vi "Append First Packet 26_01_18.vi"(4 "Movement Correction":bool, 6 "Repeat Scan":i32, 7 "MAC Address":string, 8 "Ny":i32, 9 "Nx":i32, 10 "Packets":string[](array[string]), 11 "AOL_Globals":T1={"Imaging Protocol"=enum."AOL Z-Stack", "Number of POI"=0, "Number of Miniscans"=0, "Number of Trials"=0, "Number of Cycles "=0, "# Averaged Frames"=0, "Laser power (%)"=0, "Pockels (V)"=0.0, "Acquisition Length (sec)"=0.0, "Fill time (us)"=0.0, "POI Dwell time (us)"=0.0, "Miniscan Dwell time per pixel (us)"=0.0, "PMT 1"=0.0, "PMT 2"=0.0, "Back Apperture (mA)"=0.0, "Frame Size"=0, "Center Frequency"=0.0, "Field of View (norm)"=0.0, "DwellTime (us)"=0.0, "Wavelength (nm)"=0.0, "Zoom"=0.0, "AOL Z"=0.0, "AOL Mode"=enum."Raster", "GridXY"=0.0, "GridZ"=0.0, "TriggerPeriod (sec)"=0.0, "Number of Pixels in Miniscan"=0, "Experiment folder path"=path "", "X centre"=0.0, "Y centre"=0.0, "Angle (degrees)"=0.0, "Plane Mode"=0, "Threshold"=[], "Regenerate Chirps"=FALSE, "Rectangle ROI length (pixels)"=0, "Rectangle ROI height (pixels)"=0, "AOD fill"=4900, "StartupDelay"=0, "Samples Wait after Trigger"=5080, "Slip Cycle"=600000, "Add Cycle"=TRUE, "Functional Mode"=enum."Point", "Z Start"=0.0, "Z Stop"=0.0, "# Planes"=0, "Total Pixels"=0, "Variable Miniscan Pixels"=[], "Use Variable Length"=FALSE, "Use Variable Resolution"=FALSE, "Laser power (%) at Z Start"=0, "Laser power (%) at Z Stop"=0, "Ref Z Step"=0, "Ref Dwell Time (us)"=0.0, "Field of View (um)"=175.0} {"Plane Mode" items=["XY Plane", "XZ Plane", "YZ Plane", "arbitraryplane"]; "Frame Size" items=["100X100"=100, "128X128"=128, "200X200"=200, "256X256"=256, "512X512"=512, "1024x1024"=1024, "2048x2048"=2048]; "Back Apperture (mA)" format="%#.6g"; "Pockels (V)" format="%#.6g"; "PMT 2" format="%#.6g"; "PMT 1" format="%#.6g"; "Angle (degrees)" format="%#.6g"; "POI Dwell time (us)" format="%#.6g"}) -> (0 "Repeat":i32, 2 "HexPackets":string[](array[string]), 3 "Total Packets":i32)   [LabVIEW 2020]
uses:
  Typedefs/Imaging Protocols enum.ctl
  Typedefs/Controls/AOL_Globals.ctl
  Typedefs/AOL modes.ctl
  Typedefs/Plane Mode.ctl
  Typedefs/Frame Size.ctl
  Typedefs/Functional Mode.ctl
panel:
  # "RE-ENTRANT"
  # "SUB-ROUTINE"
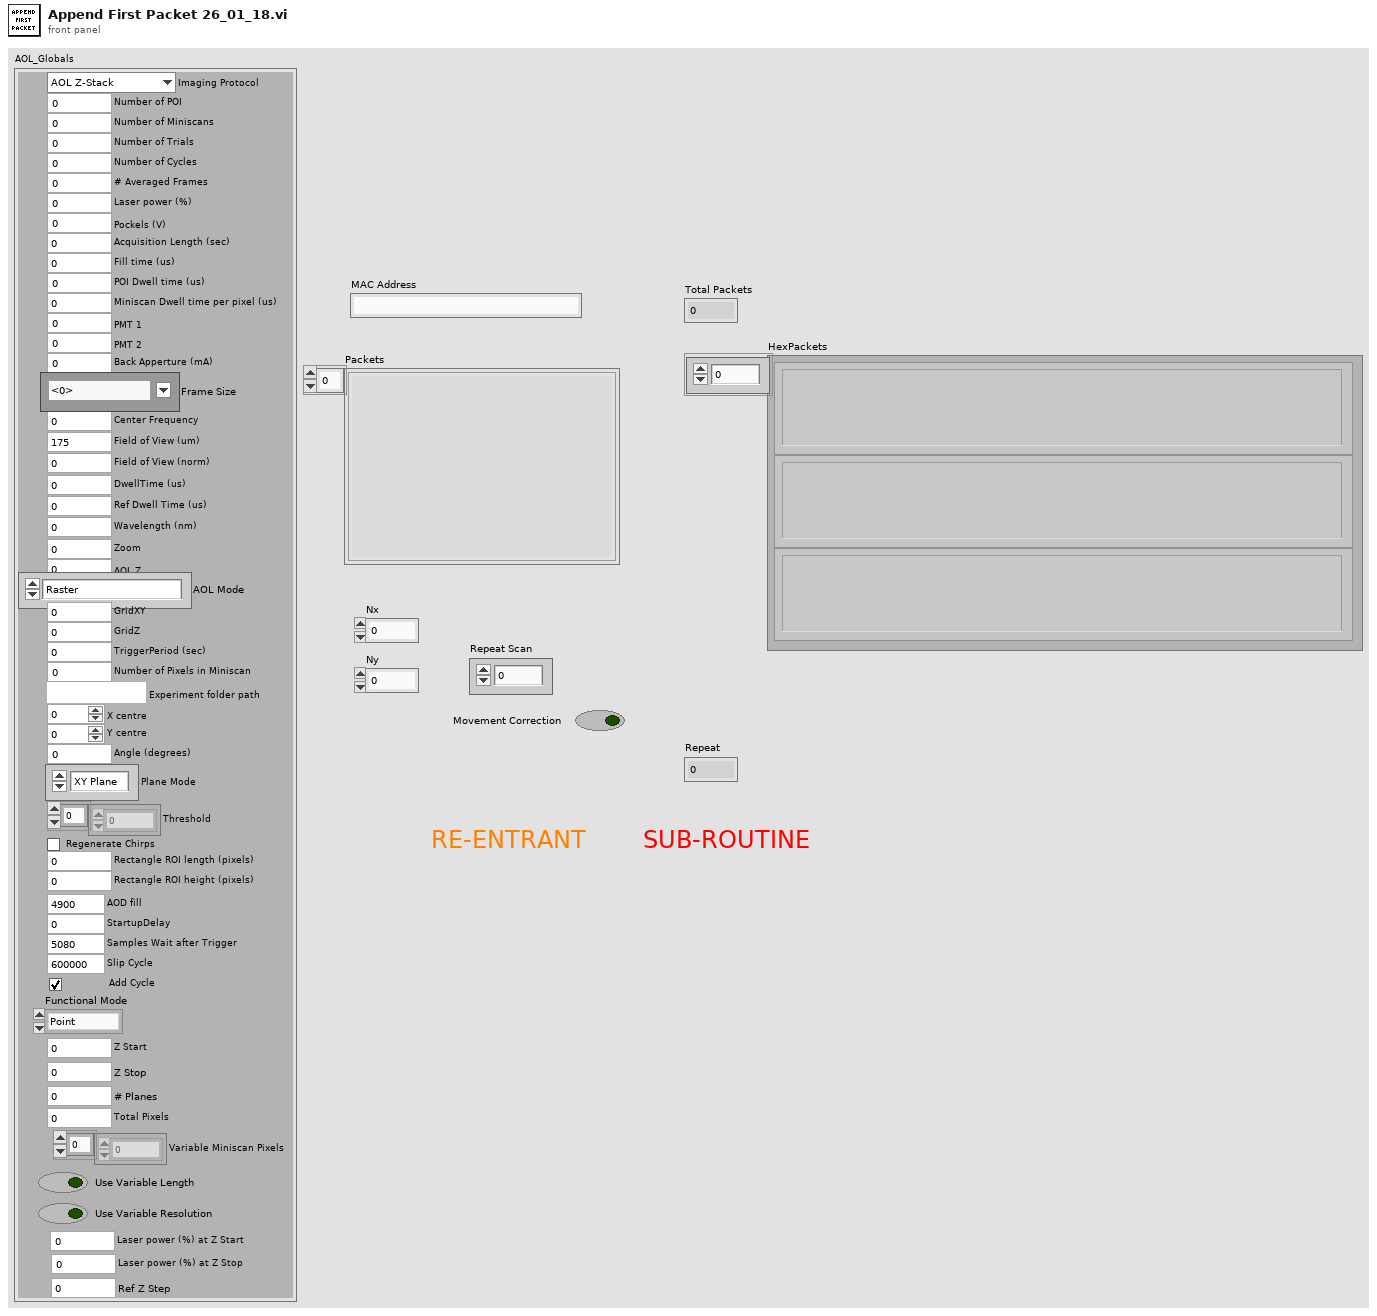
[diagram p1: front panel]
types:
  T1 = typedef "AOL_Globals.ctl" = cluster{"Imaging Protocol":T2, "Number of POI":u16, "Number of Miniscans":u16, "Number of Trials":u16, "Number of Cycles ":u64, "# Averaged Frames":u16, "Laser power (%)":u8, "Pockels (V)":dbl, "Acquisition Length (sec)":dbl, "Fill time (us)":dbl, "POI Dwell time (us)":dbl, "Miniscan Dwell time per pixel (us)":dbl, "PMT 1":dbl, "PMT 2":dbl, "Back Apperture (mA)":dbl, "Frame Size":T3, "Center Frequency":dbl, "Field of View (norm)":dbl, "DwellTime (us)":dbl, "Wavelength (nm)":dbl, "Zoom":dbl, "AOL Z":dbl, "AOL Mode":T4, "GridXY":dbl, "GridZ":dbl, "TriggerPeriod (sec)":dbl, "Number of Pixels in Miniscan":u16, "Experiment folder path":path, "X centre":dbl, "Y centre":dbl, "Angle (degrees)":dbl, "Plane Mode":T5, "Threshold":u16[], "Regenerate Chirps":bool, "Rectangle ROI length (pixels)":u16, "Rectangle ROI height (pixels)":u16, "AOD fill":u16, "StartupDelay":i32, "Samples Wait after Trigger":u16, "Slip Cycle":u32, "Add Cycle":bool, "Functional Mode":T6, "Z Start":dbl, "Z Stop":dbl, "# Planes":i32, "Total Pixels":i32, "Variable Miniscan Pixels":u16[], "Use Variable Length":bool, "Use Variable Resolution":bool, "Laser power (%) at Z Start":u8, "Laser power (%) at Z Stop":u8, "Ref Z Step":i8, "Ref Dwell Time (us)":dbl, "Field of View (um)":dbl}
  T2 = typedef "Imaging Protocols enum.ctl" = enum16{"AOL Z-Stack", "Motor Z Stack", "Functional Acquisition", "Single Plane Acquisition", "Volume Acquisition", "Live Imaging", "Live Plane Imaging", "Live Volume Imaging"}
  T3 = typedef "Frame Size.ctl" = u16
  T4 = typedef "AOL modes.ctl" = enum16{"Raster", "Structural", "Pointing", "Mini Scan", "Alignment"}
  T5 = typedef "Plane Mode.ctl" = u16
  T6 = typedef "Functional Mode.ctl" = enum16{"Point", "Line", "Patch", "Plane", "Volume"}
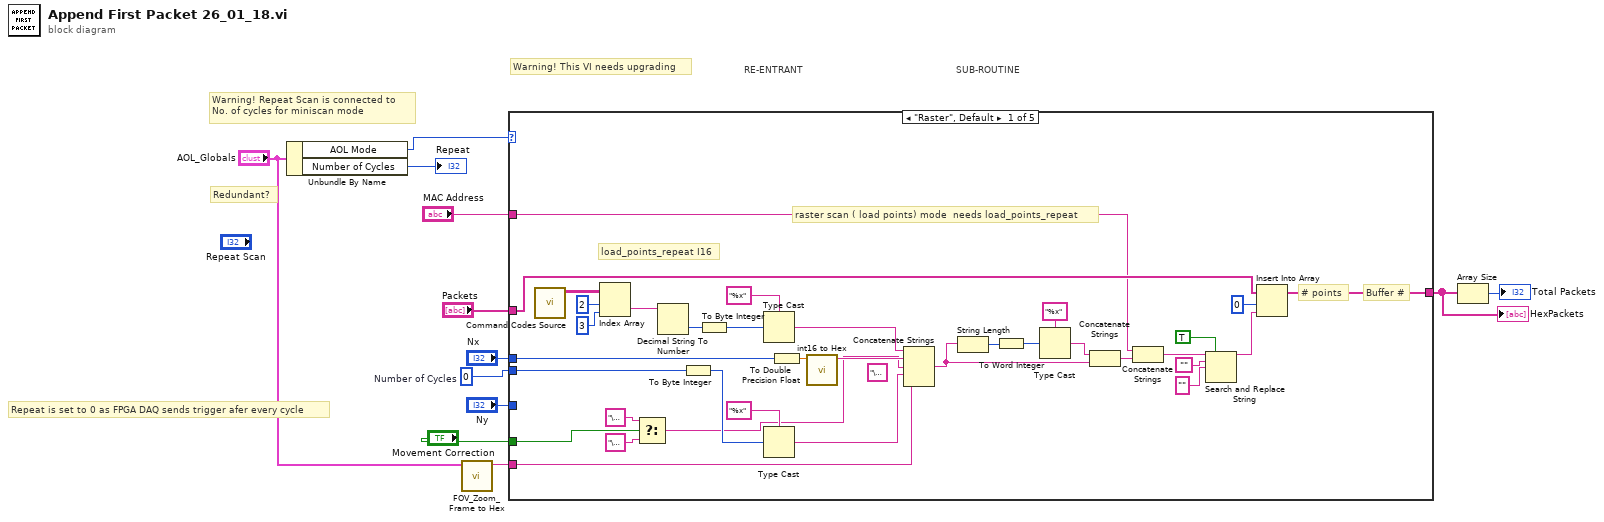
[diagram p0: block diagram]
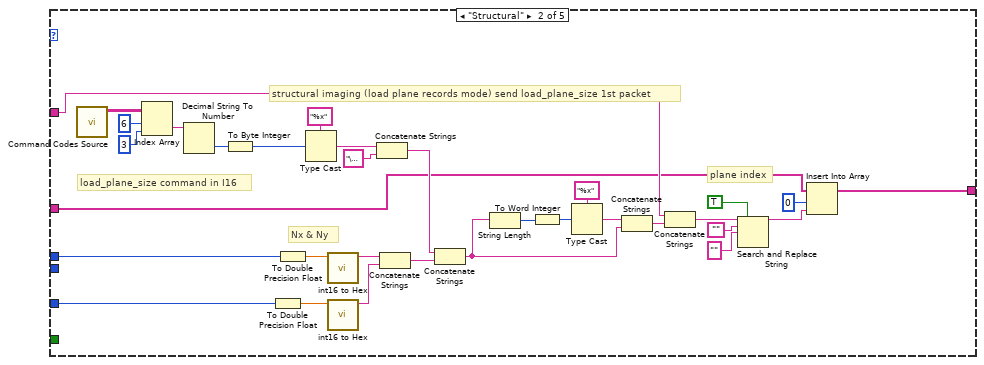
[diagram p2: hidden frame]
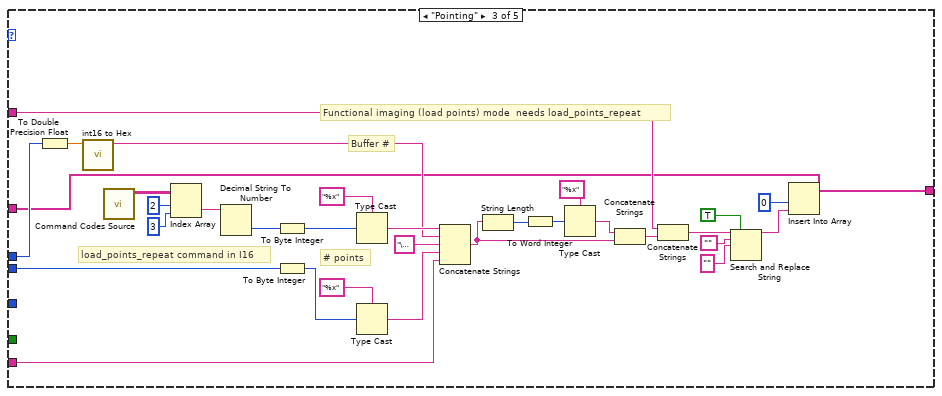
[diagram p3: hidden frame]
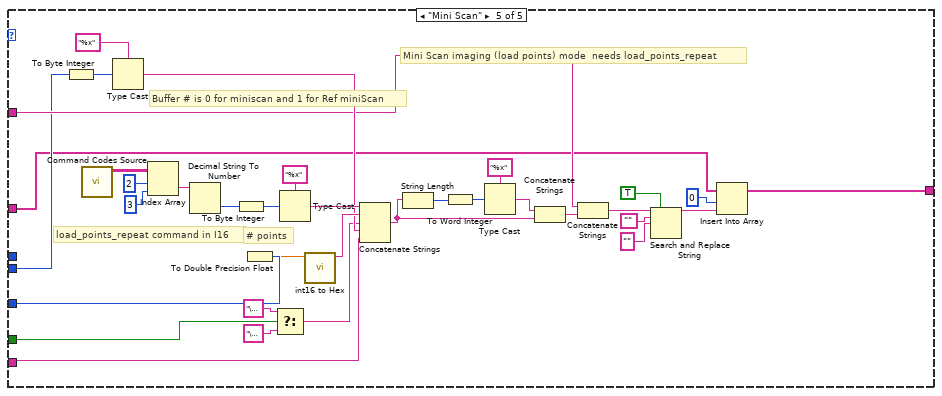
[diagram p5: hidden frame]
diagram:
  w3 = u16 0  # Number of Cycles
  # "SUB-ROUTINE"
  # "RE-ENTRANT"
  # "Repeat is set to 0 as FPGA DAQ sends trigger afer every cycle"
  # "Warning! This VI needs upgrading"
  # "Redundant?"
  # "Warning! Repeat Scan is connected to \nNo. of cycles for miniscan mode"
  n1 = Unbundle By Name("AOL_Globals") -> ("AOL Mode"=w9:T4, "Number of Cycles"=→"Repeat":u64)
  n2 = call "FOV_Zoom_Frame to Hex.vi"("AOL_Globals"="AOL_Globals") -> ("FOV-Zoom-FrameSize Hex"=w1:string)  [unwired: 10 in]
  n3 = case shown="\"Raster\", Default" w9 {
    tunnel: [w24 w52 w88 w112 w123] -> w10
    tunnel: "Ny" -> [_ w56 _ _ w117]
    tunnel: "Nx" -> [w29 w55 w93 _ _]
    tunnel: w3 -> [w15 _ w87 _ w116]
    tunnel: "Packets" -> [w26 w48 w80 w112 w113]
    tunnel: "MAC Address" -> [w20 w51 w83 _ w122]
    tunnel: "Movement Correction" -> [w17 _ _ _ w118]
    tunnel: w1 -> [w13 _ w81 _ w114]
    frame "Raster", Default {
      (unwired) "\u0000" ("string")
      # "load_points_repeat I16"
      # "# points"
      # "Buffer #"
      # "raster scan ( load points) mode  needs load_points_repeat"
      n4 = call "Command Codes Source.vi"() -> ("Commands for FPGA"=w38:string[][])  [unwired: 11 in]
      n5 = Index Array(array=w38, index (row)=2 ("disabled index (row)"), index (col)=3 ("disabled index (col)")) -> (element=w32:string)
      n6 = Select(t="\u0001" ("string"), s=w17, f="\u0000" ("string")) -> (s? t:f=w16:string)
      n7 = Decimal String To Number(string=w32) -> (number=w34:i32)  [unwired: 2 in, 1 out]
      n8 = To Byte Integer(number=w15) -> (8bit integer=w22:i8)
      n9 = To Byte Integer(number=w34) -> (8bit integer=w33:i8)
      n10 = Type Cast(type="%x", x=w33) -> (*(type *) &x=w31:string)
      n11 = Type Cast(type="%x", x=w22) -> (*(type *) &x=w21:string)
      n12 = To Double Precision Float(number=w29) -> (double precision float=w14:dbl)
      n13 = call "int16 to Hex.vi"("number"=w14) -> ("Hex string"=w28:string)  [unwired: 10 in]
      n14 = Concatenate Strings(w31, w28, w16, w21, w13) -> (w30:string)
      n15 = String Length(string=w30) -> (length=w44:i32)
      n16 = To Word Integer(number=w44) -> (16bit integer=w39:i16)
      n17 = Type Cast(type="%x", x=w39) -> (*(type *) &x=w46:string)
      n18 = Concatenate Strings(w46, w30) -> (w47:string)
      n19 = Concatenate Strings(w20, w47) -> (w43:string)
      n20 = Search and Replace String(replace all?=TRUE ("replace all? (F)"), input string=w43, search string="", replace string="" ("replace string (\"\")")) -> (result string=w25:string)  [unwired: 4 in, 3 out]
      n21 = Insert Into Array(array=w26, index=0, new element=w25) -> (w24:string[])
    }
    frame "Structural" {
      # "load_plane_size command in I16"
      # "Nx & Ny"
      # "plane index"
      # "structural imaging (load plane records mode) send load_plane_size 1st packet"
      n22 = call "Command Codes Source.vi"() -> ("Commands for FPGA"=w70:string[][])  [unwired: 11 in]
      n23 = Index Array(array=w70, index (row)=6 ("disabled index (row)"), index (col)=3 ("disabled index (col)")) -> (element=w64:string)
      n24 = Decimal String To Number(string=w64) -> (number=w66:i32)  [unwired: 2 in, 1 out]
      n25 = To Byte Integer(number=w66) -> (8bit integer=w65:i8)
      n26 = To Double Precision Float(number=w56) -> (double precision float=w49:dbl)
      n27 = To Double Precision Float(number=w55) -> (double precision float=w50:dbl)
      n28 = Type Cast(type="%x", x=w65) -> (*(type *) &x=w63:string)
      n29 = call "int16 to Hex.vi"("number"=w50) -> ("Hex string"=w60:string)  [unwired: 10 in]
      n30 = call "int16 to Hex.vi"("number"=w49) -> ("Hex string"=w59:string)  [unwired: 10 in]
      n31 = Concatenate Strings(w63, "\u0000" ("string")) -> (w61:string)
      n32 = Concatenate Strings(w60, w59) -> (w58:string)
      n33 = Concatenate Strings(w61, w58) -> (w57:string)
      n34 = String Length(string=w57) -> (length=w76:i32)
      n35 = To Word Integer(number=w76) -> (16bit integer=w71:i16)
      n36 = Type Cast(type="%x", x=w71) -> (*(type *) &x=w78:string)
      n37 = Concatenate Strings(w78, w57) -> (w79:string)
      n38 = Concatenate Strings(w51, w79) -> (w75:string)
      n39 = Search and Replace String(replace all?=TRUE ("replace all? (F)"), input string=w75, search string="", replace string="" ("replace string (\"\")")) -> (result string=w53:string)  [unwired: 4 in, 3 out]
      n40 = Insert Into Array(array=w48, index=0, new element=w53) -> (w52:string[])
    }
    frame "Pointing" {
      # "load_points_repeat command in I16"
      # "# points"
      # "Buffer #"
      # "Functional imaging (load points) mode  needs load_points_repeat"
      n41 = To Double Precision Float(number=w93) -> (double precision float=w82:dbl)
      n42 = call "int16 to Hex.vi"("number"=w82) -> ("Hex string"=w92:string)  [unwired: 10 in]
      n43 = call "Command Codes Source.vi"() -> ("Commands for FPGA"=w102:string[][])  [unwired: 11 in]
      n44 = Index Array(array=w102, index (row)=2 ("disabled index (row)"), index (col)=3 ("disabled index (col)")) -> (element=w96:string)
      n45 = Decimal String To Number(string=w96) -> (number=w98:i32)  [unwired: 2 in, 1 out]
      n46 = To Byte Integer(number=w98) -> (8bit integer=w97:i8)
      n47 = To Byte Integer(number=w87) -> (8bit integer=w85:i8)
      n48 = Type Cast(type="%x", x=w97) -> (*(type *) &x=w95:string)
      n49 = Type Cast(type="%x", x=w85) -> (*(type *) &x=w84:string)
      n50 = Concatenate Strings(w95, w92, "\u0000" ("string"), w84, w81) -> (w94:string)
      n51 = String Length(string=w94) -> (length=w108:i32)
      n52 = To Word Integer(number=w108) -> (16bit integer=w103:i16)
      n53 = Type Cast(type="%x", x=w103) -> (*(type *) &x=w110:string)
      n54 = Concatenate Strings(w110, w94) -> (w111:string)
      n55 = Concatenate Strings(w83, w111) -> (w107:string)
      n56 = Search and Replace String(replace all?=TRUE ("replace all? (F)"), input string=w107, search string="", replace string="" ("replace string (\"\")")) -> (result string=w89:string)  [unwired: 4 in, 3 out]
      n57 = Insert Into Array(array=w80, index=0, new element=w89) -> (w88:string[])
    }
    frame "Alignment" {
      # "alignment mode is load single frquency"
    }
    frame "Mini Scan" {
      # "load_points_repeat command in I16"
      # "# points"
      # "Buffer # is 0 for miniscan and 1 for Ref miniScan"
      # "Mini Scan imaging (load points) mode  needs load_points_repeat"
      n58 = To Byte Integer(number=w116) -> (8bit integer=w125:i8)
      n59 = call "Command Codes Source.vi"() -> ("Commands for FPGA"=w138:string[][])  [unwired: 11 in]
      n60 = Type Cast(type="%x", x=w125) -> (*(type *) &x=w124:string)
      n61 = Index Array(array=w138, index (row)=2 ("disabled index (row)"), index (col)=3 ("disabled index (col)")) -> (element=w132:string)
      n62 = Decimal String To Number(string=w132) -> (number=w134:i32)  [unwired: 2 in, 1 out]
      n63 = To Byte Integer(number=w134) -> (8bit integer=w133:i8)
      n64 = To Double Precision Float(number=w117) -> (double precision float=w115:dbl)
      n65 = Select(t="\u0001" ("string"), s=w118, f="\u0000" ("string")) -> (s? t:f=w119:string)
      n66 = Type Cast(type="%x", x=w133) -> (*(type *) &x=w131:string)
      n67 = call "int16 to Hex.vi"("number"=w115) -> ("Hex string"=w129:string)  [unwired: 10 in]
      n68 = Concatenate Strings(w131, w129, w119, w124, w114) -> (w130:string)
      n69 = String Length(string=w130) -> (length=w144:i32)
      n70 = To Word Integer(number=w144) -> (16bit integer=w139:i16)
      n71 = Type Cast(type="%x", x=w139) -> (*(type *) &x=w146:string)
      n72 = Concatenate Strings(w146, w130) -> (w147:string)
      n73 = Concatenate Strings(w122, w147) -> (w143:string)
      n74 = Search and Replace String(replace all?=TRUE ("replace all? (F)"), input string=w143, search string="", replace string="" ("replace string (\"\")")) -> (result string=w127:string)  [unwired: 4 in, 3 out]
      n75 = Insert Into Array(array=w113, index=0, new element=w127) -> (w123:string[])
    }
  }
  "HexPackets" <- w10
  n76 = Array Size(array=w10) -> (size(s)=→"Total Packets":i32)
